vi "power Function Derivative.vi"() -> ()   [LabVIEW 2017]
panel:
  out "Output Cluster":cluster{"X":dbl[], "Y":dbl[]} {"Y" format="%.6g"}
  out "XY Graph":cluster{dbl[], dbl[]}(graph)
  in  "Digitizing Parameters":T1={"Number of Samples"=100, "Lower Limit"=0.0, "Upper Limit"=1.0}
  in  "Function Parameters":cluster{"Prefactor":dbl, "Power":dbl}={"Prefactor"=3.0, "Power"=2.0}
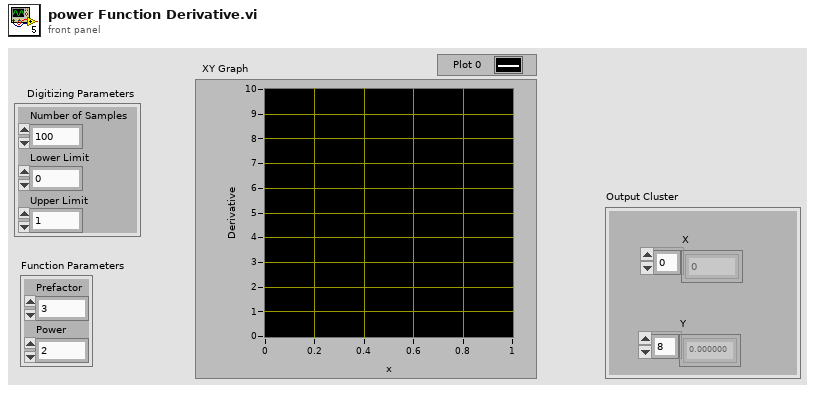
[diagram p1: front panel]
types:
  T1 = cluster{"Number of Samples":i32, "Lower Limit":dbl, "Upper Limit":dbl}
  T2 = cluster{"X Array":dbl[], "Y Array":dbl[], "delta_x":dbl}
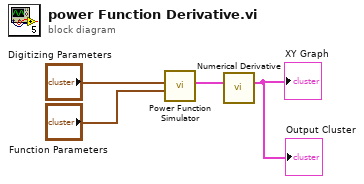
[diagram p0: block diagram]
diagram:
  n1 = call "Power Function Simulator.vi"("Function Parameters"="Function Parameters", "Digitizing Parameters"="Digitizing Parameters") -> ("Output Cluster"=w2:T2)  [unwired: 9 in]
  n2 = call "Numerical Derivative.vi"("Output Cluster"=w2) -> ("Cluster"=→"Output Cluster" →"XY Graph":cluster{"Array Without Endpoints":dbl[], dbl[]})  [unwired: 10 in]
